vi "Add Nested Enqueuer.vi"(8 "error in":errorcluster, 9 "Enq":refnum<class "Message Enqueuer.lvclass">, 10 "Ident":string, 11 "Series Actor in":refnum<class "Series Actor.lvclass">) -> (0 "error out":errorcluster, 3 "Series Actor out":refnum<class "Series Actor.lvclass">)   [LabVIEW 2024, in "Series Actor.lvlib" / "Series Actor.lvclass"]
uses:
  Series Actor.lvclass
  <vilib>/ActorFramework/Message Enqueuer/Message Enqueuer.lvclass
  Series Actor.lvclass/Series Actor.ctl
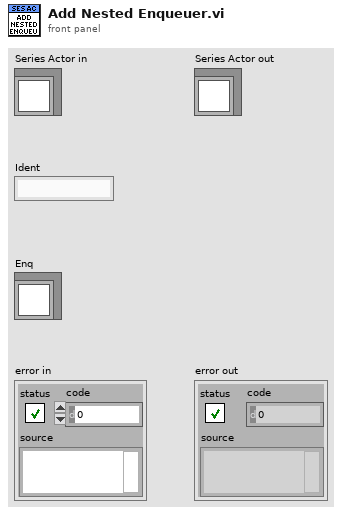
[diagram p1: front panel]
types:
  T1 = map{string, refnum<class "Message Enqueuer.lvclass">}
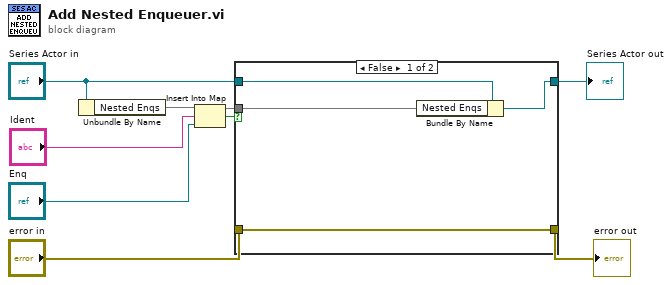
[diagram p0: block diagram]
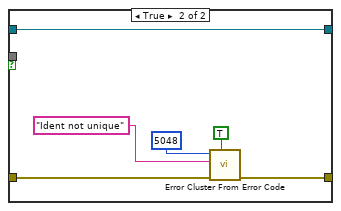
[diagram p2: hidden frame]
diagram:
  n1 = Unbundle By Name("Series Actor in") -> ("Nested Enqs"=w9:T1)
  n2 = Insert Into Map(map in=w9, key="Ident", value="Enq") -> (map out=w4:T1, key already included?=w7:bool)  [unwired: 1 out]
  n3 = case shown="False" w7 {
    tunnel: "error in" -> [w10 w19]
    tunnel: [w10 w15] -> w5
    tunnel: w4 -> [w12 _]
    tunnel: "Series Actor in" -> [w13 w14]
    tunnel: [w11 w14] -> w2
    frame False {
      n4 = Bundle By Name(cluster=w13, "Nested Enqs"=w12) -> (w11:refnum<class "Series Actor.lvclass">)
    }
    frame True {
      n5 = call <vilib>:"Error Cluster From Error Code.vi"("show call chain? (False)"=TRUE, "error in (no error)"=w19, "error message (\"\")"="Ident not unique" ("error message (\"\")"), "error code (0)"=5048) -> ("error out"=w15:errorcluster)  [unwired: 5 in]
    }
  }
  "error out" <- w5
  "Series Actor out" <- w2
